vi "Polarity Analysis.vi"(3 "error in (no error)":errorcluster, 5 "Raw Signals":waveform(dbl)[](array[waveform])) -> (0 "error out":errorcluster, 2 "Signal Integrations":dbl[](array[numeric]))   [LabVIEW 2013, in "Breakdown Acoustics Controls.lvlib"]
uses:
  Breakdown Acoustics Controls.lvlib
panel:
  in  "Time Difference\nThreshold (ms)":dbl(slide)=0.1 scale=0.0..1.0
  in  "Integration Probe\nLevel (V ms)":dbl(slide)=0.001 scale=0.0..0.01
  out "Upstream\nBreakdown":bool
  out "Downstream\nBreakdown":bool
  out "Average Time Difference":dbl
  out "Polarity Voltage Threshold Times":dbl[](graph)
  out "Signal Integrations vs. Time":dynamicdata(graph)
  out "Signal Integrations":dbl[](graph)
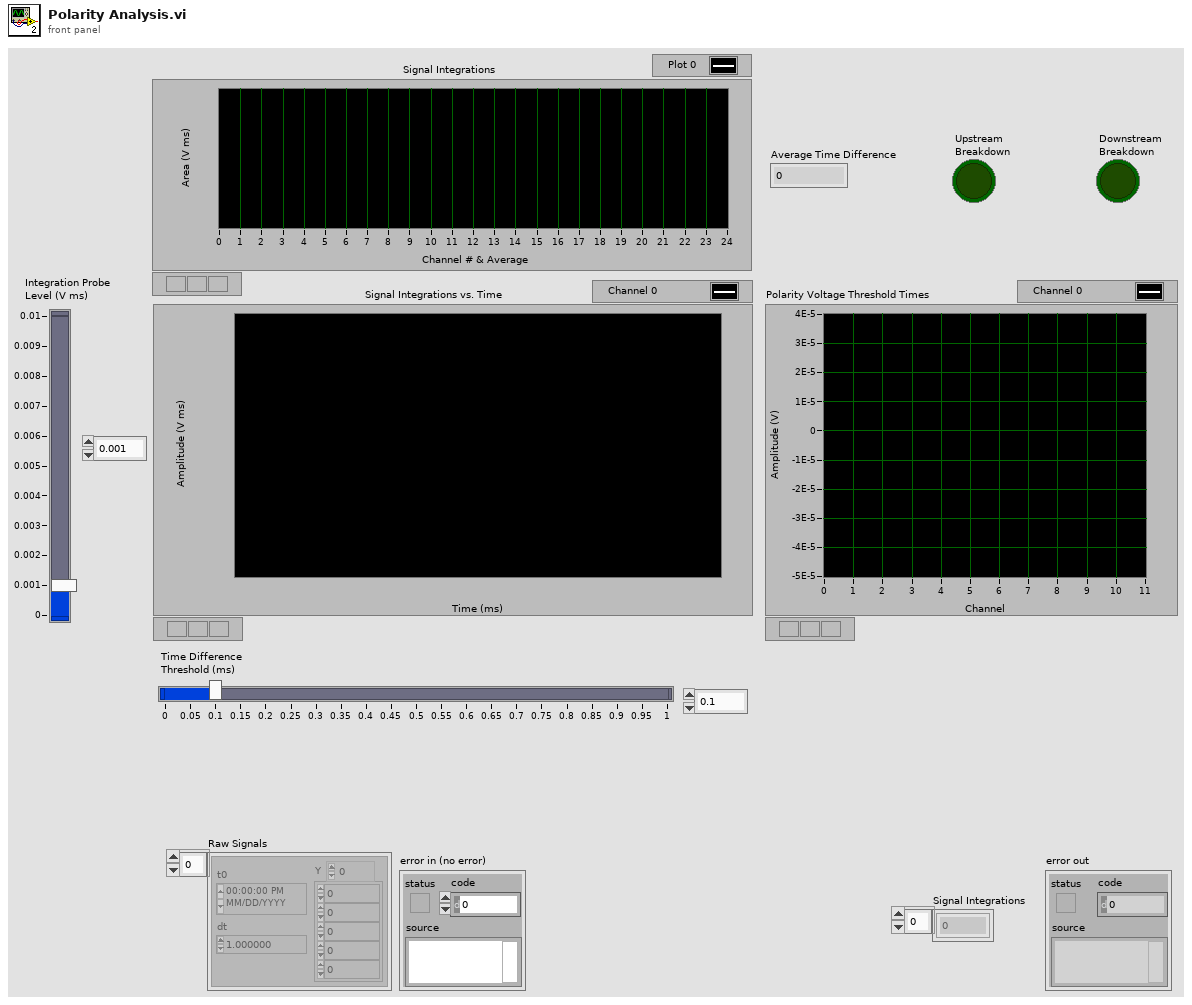
[diagram p1: front panel]
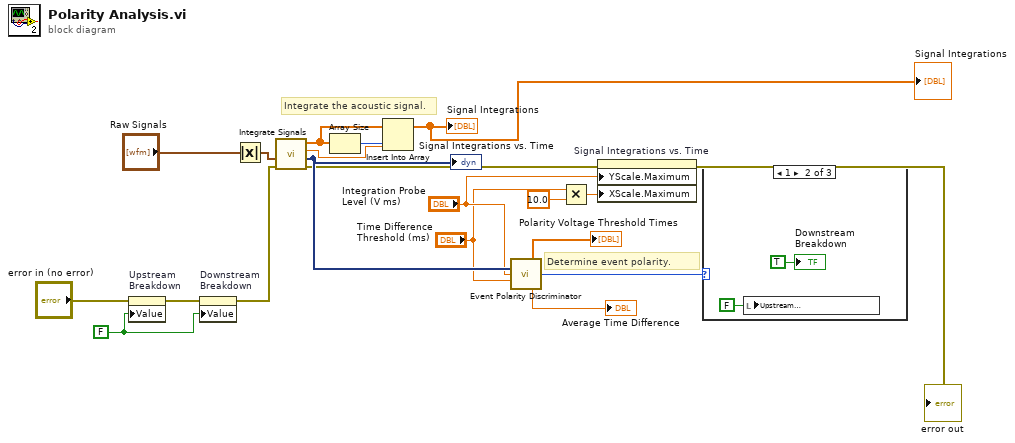
[diagram p0: block diagram]
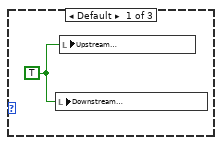
[diagram p2: hidden frame]
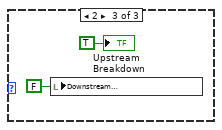
[diagram p3: hidden frame]
diagram:
  w1 = FALSE ("Upstream\nBreakdown")
  # "Determine event polarity."
  # "Integrate the acoustic signal."
  n1 = property on="Upstream\nBreakdown" class="Bool (strict)"(error in="error in (no error)", "Value"=w1) -> (error out=w4:errorcluster)  [unwired: 1 in, 1 out]
  n2 = property on="Downstream\nBreakdown" class="Bool (strict)"(error in=w4, "Value"=w1) -> (error out=w2:errorcluster)  [unwired: 1 in, 1 out]
  n3 = Absolute Value(x="Raw Signals") -> (abs(x)=w11:waveform(dbl)[])
  n4 = call "Integrate Signals.vi"("error in (no error)"=w2, "Signals"=w11) -> ("error out"=→"error out":errorcluster, "Integration vs. Time"=w14:dynamicdata, "Average Integration Value"=w18:dbl, "Integration Values"=w13:dbl[])  [unwired: 6 in]
  "Signal Integrations vs. Time" <- w14
  n5 = Array Size(array=w13) -> (size(s)=w19:i32)
  n6 = Insert Into Array(array=w13, index=w19, new element=w18) -> (→"Signal Integrations" →"Signal Integrations":dbl[])
  n7 = call "Event Polarity Discriminator.vi"("Integrations vs. Time"=w14, "Integration Level (V ms)"="Integration Probe\nLevel (V ms)", "Time Difference Threshold (ms)"="Time Difference\nThreshold (ms)") -> ("Time Differences"=→"Polarity Voltage Threshold Times":dbl[], "Event Polarity"=w15:u32, "Average Time Diference"=→"Average Time Difference":dbl)  [unwired: 10 in]
  n8 = Multiply(x="Time Difference\nThreshold (ms)", y=10.0) -> (x*y=w9:dbl)
  n9 = property on="Signal Integrations vs. Time" class="WFGraph (strict)"("YScale.Maximum"="Integration Probe\nLevel (V ms)", "XScale.Maximum"=w9) -> ()  [unwired: 2 in, 2 out]
  n10 = case shown="1" w15 {
    frame Default {
      w20 = TRUE ("Upstream\nBreakdown")
      n11 = local write "Downstream\nBreakdown"(w20) -> ()
      n12 = local write "Upstream\nBreakdown"(w20) -> ()
    }
    frame 1 {
      n13 = local write "Upstream\nBreakdown"(FALSE ("Upstream\nBreakdown")) -> ()
      "Downstream\nBreakdown" <- TRUE ("Downstream\nBreakdown")
    }
    frame 2 {
      n14 = local write "Downstream\nBreakdown"(FALSE ("Downstream\nBreakdown")) -> ()
      "Upstream\nBreakdown" <- TRUE ("Upstream\nBreakdown")
    }
  }
